vi "MACBIN Copy Fork To File__ogtk.vi"(4 "file size":i32, 5 "error out":errorcluster, 7 "fork Refnum":refnum<file>, 8 "macbinary Refnum":refnum<file>) -> (0 "error out":errorcluster, 2 "filename out":path, 3 "macbinary Refnum out":refnum<file>)   [LabVIEW 2016]
panel:
  # "Please visit http://www.OpenG.org to learn about the\nOpen Source LabVIEW software movement.\n\nNOTICE -- YOU MUST LEAVE THIS NOTICE IN PLACE.  PER THE TERMS OF THE LICENSE BELOW, YOU MAY SUBLICENSE THIS SOFTWARE \nIN ANY WAY THAT DOES NOT CONFLICT WITH THIS LICENSE.\n\n### BSD License (http://www.opensource.org/licenses/bsd-license.php) Begin ###\n \nCopyright (C) 2002 Christophe Salzmann christophe.salzmann@epfl.ch\nCopyright (C) 2002 Rolf Kalbermatter rolf.kalbermatter@citengineering.com\n\nAll rights reserved.\n\nRedistribution and use in source and binary forms, with or without modification, are permitted provided that the following conditions are met:\n\n    * Redistributions of source code must retain the above copyright notice, this list of conditions and the following disclaimer.\n    * Redistributions in binary form must reproduce the above copyright notice, this list of conditions and the following disclaimer in the \n       documentation and/or other materials provided with the distribution.\n    * Neither the name of SciWare, James Kring, Inc., nor the names of its contributors may be used to endorse or promote products derived \n       from this software without specific prior written permission.\n\nTHIS SOFTWARE IS PROVIDED BY THE COPYRIGHT HOLDERS AND CONTRIBUTORS \"AS IS\" AND ANY EXPRESS OR IMPLIED WARRANTIES, \nINCLUDING, BUT NOT LIMITED TO, THE IMPLIED WARRANTIES OF MERCHANTABILITY AND FITNESS FOR A PARTICULAR PURPOSE ARE \nDISCLAIMED. IN NO EVENT SHALL THE COPYRIGHT OWNER OR CONTRIBUTORS BE LIABLE FOR ANY DIRECT, INDIRECT, INCIDENTAL,\n SPECIAL, EXEMPLARY, OR CONSEQUENTIAL DAMAGES (INCLUDING, BUT NOT LIMITED TO, PROCUREMENT OF SUBSTITUTE GOODS OR \nSERVICES; LOSS OF USE, DATA, OR PROFITS; OR BUSINESS INTERRUPTION) HOWEVER CAUSED AND ON ANY THEORY OF LIABILITY, \nWHETHER IN CONTRACT, STRICT LIABILITY, OR TORT (INCLUDING NEGLIGENCE OR OTHERWISE) ARISING IN ANY WAY OUT OF THE USE \nOF THIS SOFTWARE, EVEN IF ADVISED OF THE POSSIBILITY OF SUCH DAMAGE.\n\n### BSD License End ###"
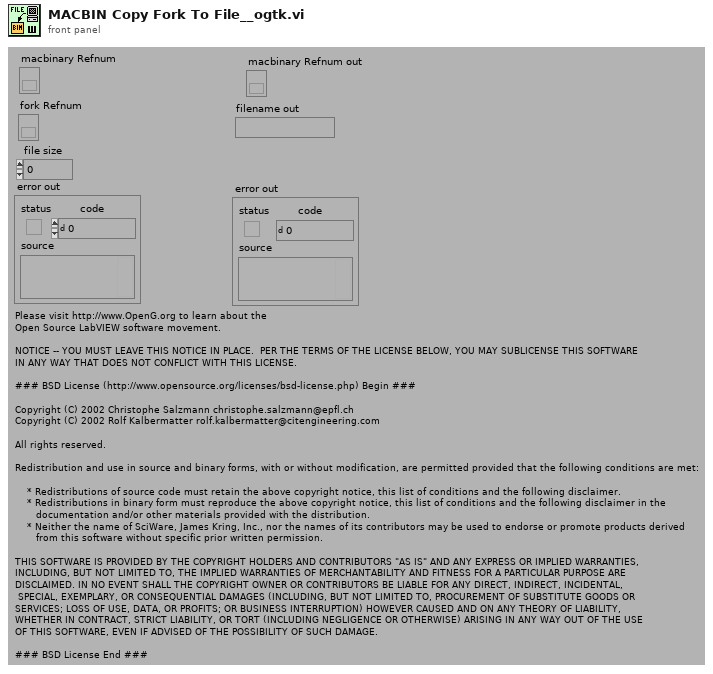
[diagram p1: front panel]
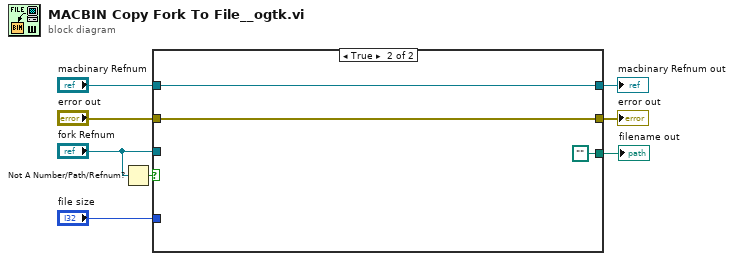
[diagram p0: block diagram]
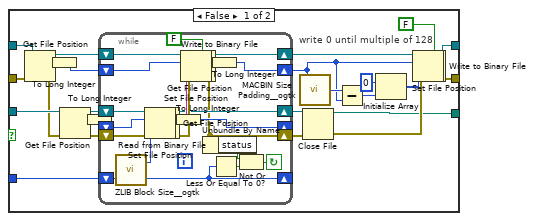
[diagram p2: hidden frame]
diagram:
  n1 = Not A Number/Path/Refnum?(number/path/refnum="fork Refnum") -> (NaN/Path/Refnum?=w1:bool)
  n2 = case shown="True" w1 {
    tunnel: "file size" -> [w35 _]
    tunnel: [w34 w66] -> w7
    tunnel: [w32 w67] -> w6
    tunnel: "fork Refnum" -> [w25 _]
    tunnel: "macbinary Refnum" -> [w21 w66]
    tunnel: "error out" -> [w18 w67]
    tunnel: [w14 path ""] -> w3
    frame False {
      # "write 0 until multiple of 128"
      n3 = Get File Position(4:w18, 7:w21) -> (0:w17:errorcluster, 2:w13:i64, 3:w19:refnum<file>)
      n4 = To Long Integer(number=w13) -> (32bit integer=w20:i32)
      n5 = Get File Position(4:w17, 7:w25) -> (0:w23:errorcluster, 2:w12:i64, 3:w24:refnum<file>)
      n6 = To Long Integer(number=w12) -> (32bit integer=w22:i32)
      n7 = while {
        shift-left: w35 -> [w53]
        shift-right: [w47] -> _
        shift-left: w24 -> [w55]
        shift-right: [w54] -> w29
        shift-left: w22 -> [w57]
        shift-right: [w56] -> _
        shift-left: w19 -> [w60]
        shift-right: [w59] -> w33
        shift-left: w23 -> [w58]
        shift-right: [w51] -> w30
        shift-left: w20 -> [w62]
        shift-right: [w61] -> w15
        stop <- w50 continue-if-true
        n8 = call <userlib>:"ZLIB Block Size__ogtk.vi"("length in"=w53) -> ("length rem"=w47:u32, "block len"=w52:u32)  [unwired: 1 in]
        n9 = Set File Position(offset (in bytes) (0)=w57, refnum=w55, error in=w58) -> (refnum out=w46:refnum<file>, error out=w45:errorcluster)  [unwired: 1 in]
        n10 = Read from Binary File(8:w45, 10:w52, 11:w46) -> (0:w43:errorcluster, 2:w64:string, 3:w44:refnum<file>)  [unwired: 3 in, 1 out]
        n11 = Get File Position(4:w43, 7:w44) -> (0:w63:errorcluster, 2:w42:i64, 3:w54:refnum<file>)
        n12 = To Long Integer(number=w42) -> (32bit integer=w56:i32)
        n13 = Set File Position(offset (in bytes) (0)=w62, refnum=w60, error in=w63) -> (refnum out=w41:refnum<file>, error out=w40:errorcluster)  [unwired: 1 in]
        n14 = Write to Binary File(file (use dialog)=w41, data=w64, error in=w40, 5:FALSE ("prepend array or string size? (T)")) -> (refnum out=w39:refnum<file>, error out=w38:errorcluster)  [unwired: 2 in, 1 out]
        n15 = Get File Position(4:w38, 7:w39) -> (0:w51:errorcluster, 2:w37:i64, 3:w59:refnum<file>)
        n16 = Unbundle By Name(w51) -> ("status"=w49:bool)
        n17 = To Long Integer(number=w37) -> (32bit integer=w61:i32)
        n18 = Less Or Equal To 0?(x=w47) -> (x <= 0?=w48:bool)
        n19 = Not Or(1:w48, 2:w49) -> (0:w50:bool)
      }
      n20 = call <userlib>:"MACBIN Size Padding__ogtk.vi"("length"=w15) -> ("padded length"=w16:i32)  [unwired: 4 in]
      n21 = Close File(refnum=w29, error in=w30) -> (path=w14:path, error out=w31:errorcluster)
      n22 = Subtract(x=w16, y=w15) -> (x-y=w28:i32)
      n23 = Initialize Array(u8 0 ("offset"), w28) -> (w26:u8[])
      n24 = Set File Position(offset (in bytes) (0)=w15, refnum=w33, error in=w31) -> (refnum out=w11:refnum<file>, error out=w10:errorcluster)  [unwired: 1 in]
      n25 = Write to Binary File(file (use dialog)=w11, data=w26, error in=w10, 5:FALSE ("prepend array or string size? (T)")) -> (refnum out=w34:refnum<file>, error out=w32:errorcluster)  [unwired: 2 in, 1 out]
    }
    frame True {
    }
  }
  "macbinary Refnum out" <- w7
  "error out" <- w6
  "filename out" <- w3
